vi "CastSpell.vi"(8 "error in (no error)":errorcluster, 11 "EnchantedMazeGame in":refnum<class "EnchantedMazeGame.lvclass">) -> (0 "error out":errorcluster, 2 "Spell":refnum<class "Spell.lvclass">, 3 "EnchantedMazeGame out":refnum<class "EnchantedMazeGame.lvclass">)   [LabVIEW 2020, in "FactoryMethod.lvlib" / "NoParametrizedFactoryMethod.lvlib" / "EnchantedMazeGame.lvclass"]
uses:
  EnchantedMazeGame.lvclass
  GoFcommonClasses/Spell/Spell.lvclass
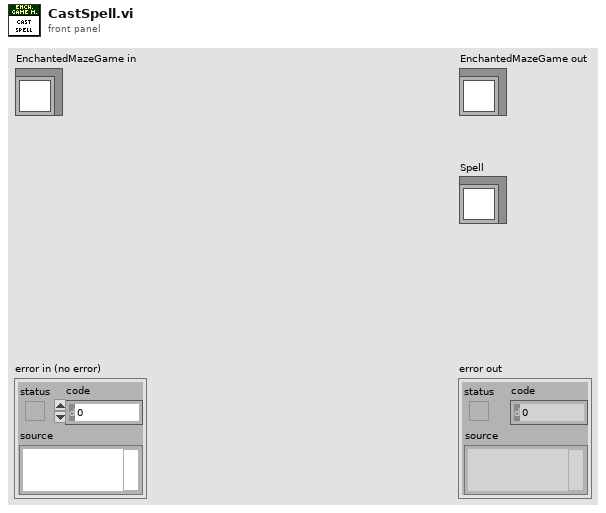
[diagram p1: front panel]
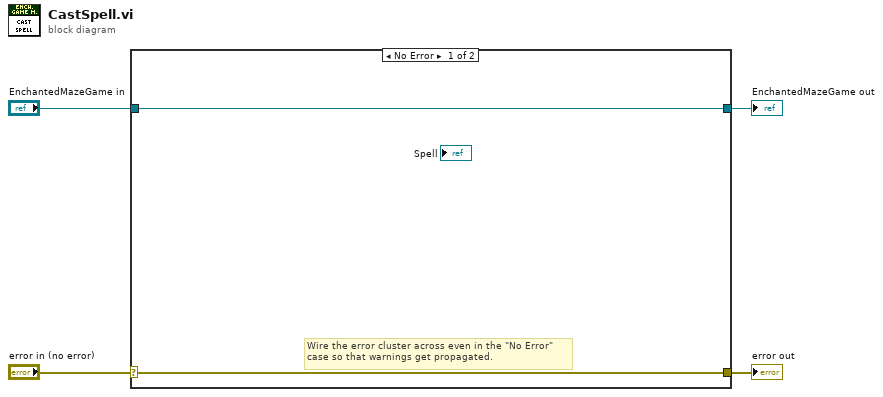
[diagram p0: block diagram]
diagram:
  n1 = case shown="No Error" "error in (no error)" {
    selector: "error in (no error)" -> [w5 w8]
    tunnel: [w5 w8] -> w3
    tunnel: [w6 w7] -> w1
    tunnel: "EnchantedMazeGame in" -> [w6 w7]
    frame No Error {
      # "Wire the error cluster across even in the \"No Error\"\ncase so that warnings get propagated."
    }
    frame Error {
    }
  }
  "error out" <- w3
  "EnchantedMazeGame out" <- w1
